vi "浮点数所在区间（利用复数）.vi"(1 "上下限数组":cluster{"上限":dbl, "下限":dbl}[](array[cluster])=[{"上限"=0.0, "下限"=-inf}, {"上限"=10.0, "下限"=0.0}, {"上限"=20.0, "下限"=10.0}, {"上限"=50.0, "下限"=20.0}], 2 "比较值":dbl) -> (0 "范围":cluster{"上限":dbl, "下限":dbl})   [LabVIEW 2012]
panel:
  out "区间索引":i32
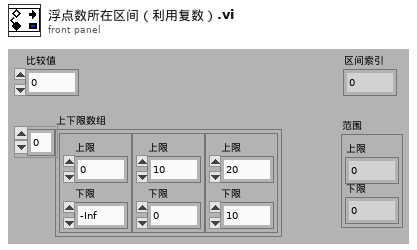
[diagram p1: front panel]
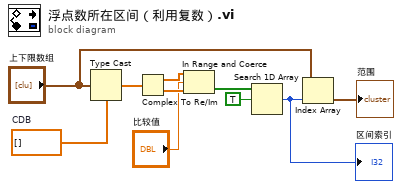
[diagram p0: block diagram]
diagram:
  w10 = cdb[] []  # CDB
  n1 = Type Cast(type=w10, x="上下限数组") -> (*(type *) &x=w9:cdb[])
  n2 = Complex To Re/Im(x + iy=w9) -> (x=w8:dbl[], y=w7:dbl[])
  n3 = In Range and Coerce(upper limit=w8, x="比较值", lower limit=w7) -> (In Range?=w5:bool[])  [unwired: 1 out]
  n4 = Search 1D Array(1D array=w5, element=TRUE ("元素")) -> (index of element=w2:i32)  [unwired: 1 in]
  "区间索引" <- w2
  n5 = Index Array(array="上下限数组", index=w2) -> (element=→"范围":cluster{"上限":dbl, "下限":dbl})
